vi "FTW-ActorExtended-Child-PoisonPill.vi"(0 "FTW-ActorExtended In":refnum<class "FTW-ActorExtended.lvclass">, 5 "Connector Name":string, 9 "Timeout":i32=100 format="%dmsec", 11 "error in":errorcluster) -> (4 "FTW-ActorExtended Out":refnum<class "FTW-ActorExtended.lvclass">, 6 "Response Header":string, 8 "Response Body":string, 10 "Timed out?":bool, 14 "Roundtrip Time":dbl format="%.6fsec", 15 "error out":errorcluster)   [LabVIEW 2013, in "FTW-ActorExtended.lvclass"]
uses:
  FTW-ActorExtended.lvclass
  Connector/FTW-ActorConnector.lvclass
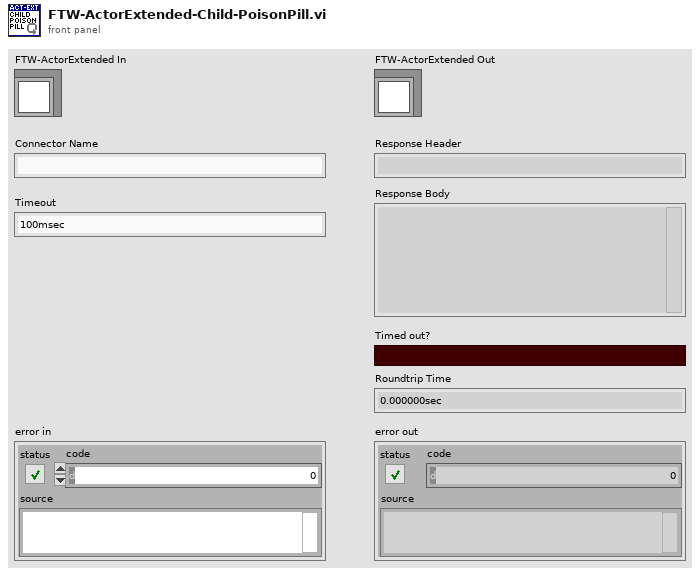
[diagram p1: front panel]
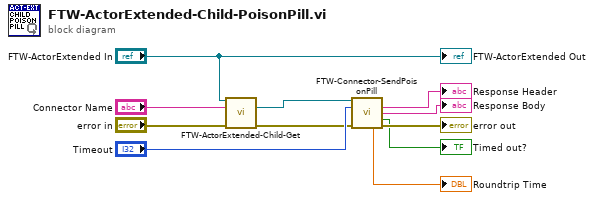
[diagram p0: block diagram]
diagram:
  n1 = call "FTW-ActorExtended-Child-Get.vi"("FTW-ActorExtended In"="FTW-ActorExtended In", "Connector Name"="Connector Name", "error in"="error in") -> ("FTW Actor Connector"=w3:refnum<class "FTW-ActorConnector.lvclass">, "error out"=w4:errorcluster)  [unwired: 10 in, 1 out]
  n2 = call-dynamic "FTW-Connector-SendPoisonPill.vi"("FTW Actor Connector"=w3, "Timeout"="Timeout", "error in"=w4) -> ("Response Header"=→"Response Header":string, "Response Body"=→"Response Body":string, "Timed out?"=→"Timed out?":bool, "Roundtrip Time"=→"Roundtrip Time":dbl, "error out"=→"error out":errorcluster)  [unwired: 7 in, 1 out]
  "FTW-ActorExtended Out" <- "FTW-ActorExtended In"
